vi "test gradient descent.vi"() -> ()   [LabVIEW 2014]
uses:
  Target Functions.ctl
  <vilib>/Analysis/NI_AALBase.lvlib
  <vilib>/vision/Image Controls.llb/IMAQ Image.ctl
  Measurements/Instrument Sequence/Instrument Sequence Notifiers.ctl
  Measurements/Save Data/SaveData Notifiers.ctl
  Autofocus Notifiers.ctl
  Tango XYZ Stage/Tango Notifications.ctl
  Camera/Camera Notifiers.ctl
  Switches and Mirrors/SwitchesMirrors Notifiers.ctl
  NGSLabspec/LabramHR Notifiers.ctl
  Newport ESP301/StressControl Notifiers.ctl
  Keithley707A/Keithley 707A Notifiers.ctl
  HP4155C/HP4155C Notifiers.ctl
  controls/IBM OptoElectroMechanics Message Handler Loop Notifiers.ctl
  support/Notifiers/Notifiers.ctl
  <vilib>/Analysis/Matrix/Datatypes/RealMatrix.ctl
  <vilib>/Analysis/Matrix/NI_Matrix.lvlib
  support/Message Queue/Message Cluster.ctl
  support/Message Queue/IBM OptoElectroMechanics Message Queue.lvlib
  support/Message Queue/All Message Queues.ctl
  Target Refnums.ctl
  AutoFocus Refnums.ctl
  <vilib>/Analysis/baseanly.llb/A x Vector.vi
  ZScan.ctl
panel:
  in  "Z Scan Parameters":T1={"Z Range"=1380.0, "Resolution"=5000.0, "Initial Direction"=enum."Up", "Descent Constant"=0.1} {"Descent Constant" min=0.0 max=1000.0 step=1.0 format="%#_2f"; "Resolution" min=0.0 max=1.0 step=0.01 format="%_2g"; "Z Range" format="%_3g"}
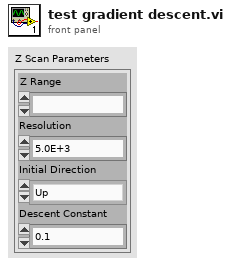
[diagram p1: front panel]
types:
  T1 = typedef "ZScan.ctl" = cluster{"Z Range":ext, "Resolution":dbl, "Initial Direction":enum16{"Up", "Down"}, "Descent Constant":dbl}
  T2 = typedef "AutoFocus Refnums.ctl" = cluster{"Instrument Status":refnum<vi>, "Matching Criteria":refnum<vi>, "Z Scan Parameters":refnum<vi>, "Distance":refnum<vi>, "Transformation Matrix":refnum<vi>, "Match and Edge":T3, "Matching Curves":refnum<vi>, "Tracking":refnum<vi>, "Focus":refnum<vi>, "Find Focus":refnum<vi>, "Set Target":refnum<vi>, "Link Stage & Camera":refnum<vi>, "Align":refnum<vi>}
  T3 = typedef "Target Refnums.ctl" = cluster{"Image":refnum<vi>, "Target":refnum<vi>, "Edge":refnum<vi>, "Target Data":refnum<vi>}
  T4 = typedef "IBM OptoElectroMechanics Message Queue.lvlib/All Message Queues.ctl" = cluster{"Message Handler Loop":refnum<queue>, "Parameter Analyzer":refnum<queue>, "Switching Matrix":refnum<queue>, "Stress Control":refnum<queue>, "Optical Spectrometer":refnum<queue>, "Switches & Mirrors":refnum<queue>, "Camera":refnum<queue>, "XYZ Stage":refnum<queue>, "AutoFocus":refnum<queue>, "Save Data":refnum<queue>, "Plot Data":refnum<queue>, "Instrument Sequence":refnum<queue>, "Strain Measurement":refnum<queue>}
  T5 = typedef "NI_Matrix.lvlib/RealMatrix.ctl" = dbl[][]
  T6 = cluster{"Match":cluster{"Position":cluster{"x":sgl, "y":sgl}, "Angle":sgl, "Scale":sgl, "Score":sgl, "Bounding Box":cluster{"x":sgl, "y":sgl}[]}, "Edge Analysis":cluster{"Mean Value":sgl, "Standard Variation":sgl, "Minimal Value":sgl, "Maximal Value":sgl, "Area (calibrated)":sgl, "Area (pixels)":i32, "%":sgl}}
  T7 = cluster{"Focus Plot":cluster{"Z (um)":dbl[], "Score":sgl[]}[], "max":sgl, "min":sgl}
  T8 = cluster{"Minimum Score":sgl, "Color Score Weight":sgl, "Minimum Contrast":i32, "Match Mode":u32, "Match Feature Mode":u32, "Subpixel Accuracy":bool, "Color Sensitivity":u32, "Search Strategy":u32}
  T9 = typedef "Notifiers.ctl" = cluster{"Message Handler Loop":T10, "Parameter Analyzer":T11, "Switching Matrix":T12, "Stress Control":T13, "Optical Spectrometer":T14, "Switches & Mirrors":T15, "Camera":T16, "XYZ Stage":T17, "AutoFocus":T18, "Save Data":T19, "Plot Data":T19, "Instrument Sequence":T20, "Strain Measurement":cluster{"Status":refnum<notifier>, "Exit":refnum<notifier>, "Ready":refnum<notifier>}}
  T10 = typedef "IBM OptoElectroMechanics Message Handler Loop Notifiers.ctl" = cluster{"Status":refnum<notifier>, "Instrument Data":refnum<notifier>, "Exit":refnum<notifier>, "Ready":refnum<notifier>}
  T11 = typedef "HP4155C Notifiers.ctl" = cluster{"Status":refnum<notifier>, "Instrument Data":refnum<notifier>, "Measurement":refnum<notifier>, "Exit":refnum<notifier>, "Ready":refnum<notifier>}
  T12 = typedef "Keithley 707A Notifiers.ctl" = cluster{"Status":refnum<notifier>, "Instrument Data":refnum<notifier>, "Measurement":refnum<notifier>, "Exit":refnum<notifier>, "Ready":refnum<notifier>}
  T13 = typedef "StressControl Notifiers.ctl" = cluster{"Status":refnum<notifier>, "Instrument Data":refnum<notifier>, "Measurement":refnum<notifier>, "Exit":refnum<notifier>, "Ready":refnum<notifier>}
  T14 = typedef "LabramHR Notifiers.ctl" = cluster{"Status":refnum<notifier>, "Instrument Data":refnum<notifier>, "Measurement":refnum<notifier>, "Exit":refnum<notifier>, "Ready":refnum<notifier>}
  T15 = typedef "SwitchesMirrors Notifiers.ctl" = cluster{"Status":refnum<notifier>, "Instrument Data":refnum<notifier>, "Exit":refnum<notifier>, "Ready":refnum<notifier>}
  T16 = typedef "Camera Notifiers.ctl" = cluster{"Status":refnum<notifier>, "Instrument Data":refnum<notifier>, "Measurement":refnum<notifier>, "Exit":refnum<notifier>, "Ready":refnum<notifier>}
  T17 = typedef "Tango Notifications.ctl" = cluster{"Status":refnum<notifier>, "Instrument Data":refnum<notifier>, "Measurement":refnum<notifier>, "Exit":refnum<notifier>, "Ready":refnum<notifier>}
  T18 = typedef "Autofocus Notifiers.ctl" = cluster{"Status":refnum<notifier>, "Instrument Data":refnum<notifier>, "Measurement":refnum<notifier>, "Exit":refnum<notifier>, "Ready":refnum<notifier>}
  T19 = typedef "SaveData Notifiers.ctl" = cluster{"Status":refnum<notifier>, "Exit":refnum<notifier>, "Ready":refnum<notifier>}
  T20 = typedef "Instrument Sequence Notifiers.ctl" = cluster{"Status":refnum<notifier>, "Instrument Data":refnum<notifier>, "Measurement":refnum<notifier>, "Exit":refnum<notifier>, "Ready":refnum<notifier>}
  T21 = typedef "IMAQ Image.ctl" = refnum<image>
  T22 = typedef "Target Functions.ctl" = enum16{"Setup Match Criteria", "Set Target", "Find Target"}
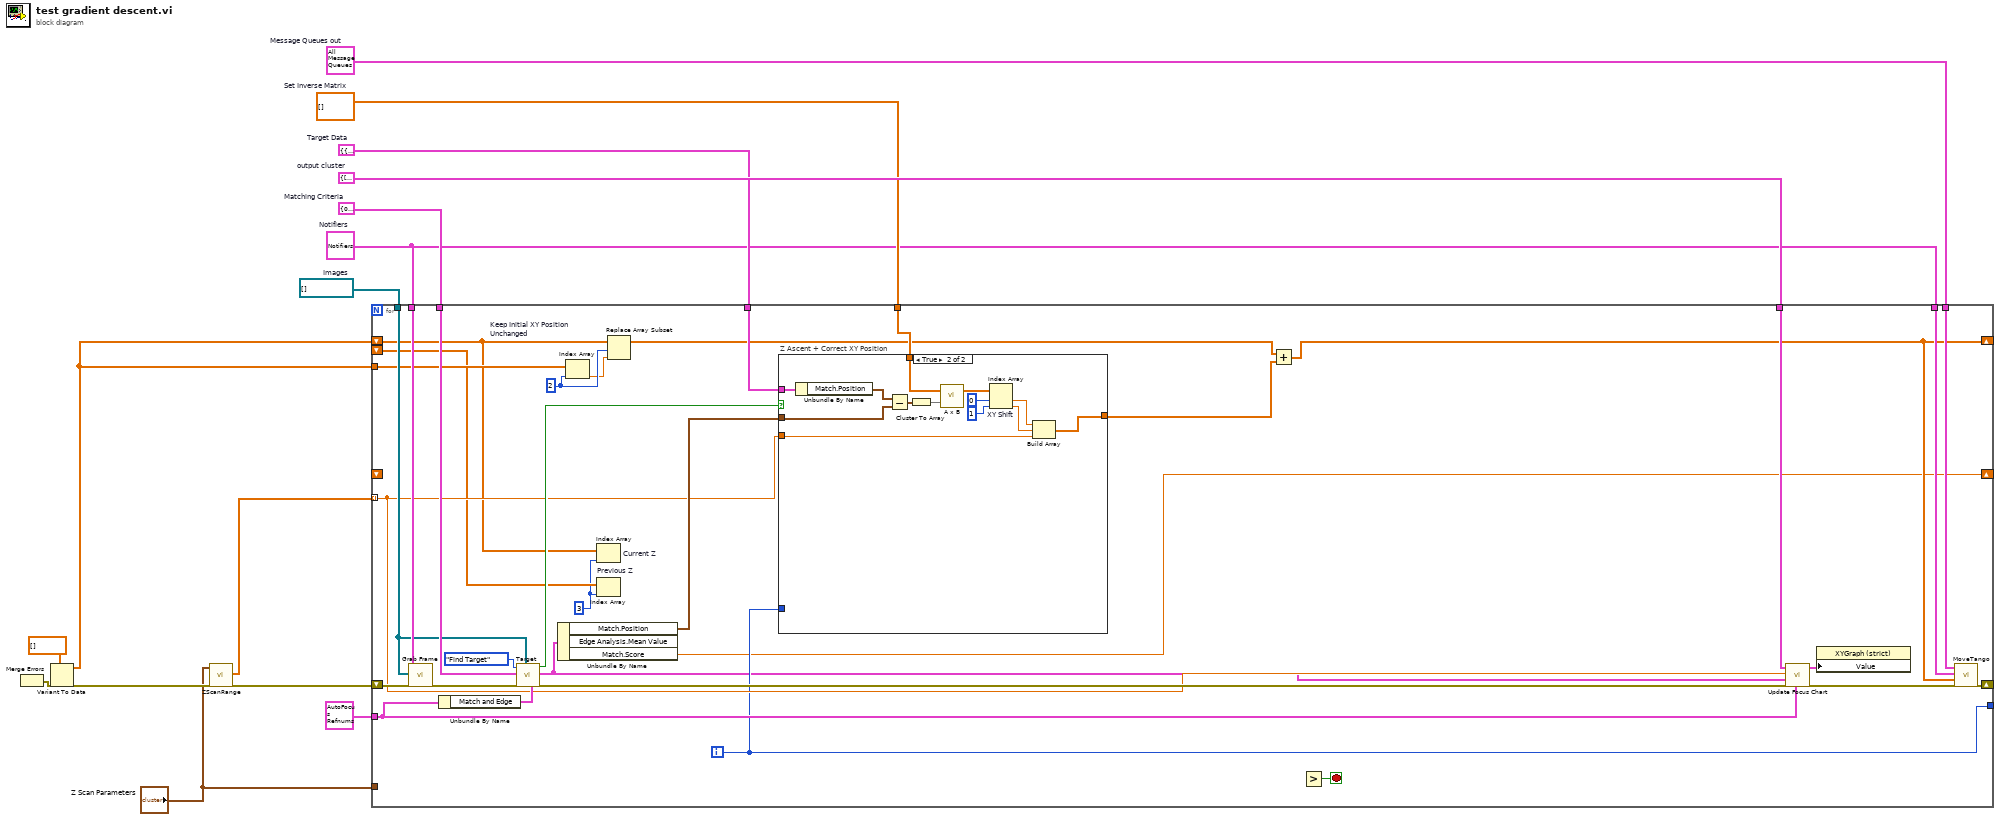
[diagram p0: block diagram]
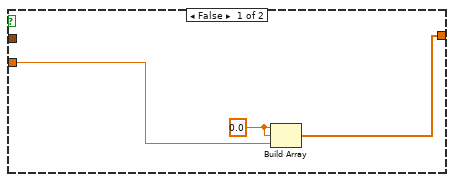
[diagram p2: hidden frame]
diagram:
  w3 = T4 {"Message Handler Loop"=refnum, "Parameter Analyzer"=refnum, "Switching Matrix"=refnum, "Stress Control"=refnum, "Optical Spectrometer"=refnum, "Switches & Mirrors"=refnum, "Camera"=refnum, "XYZ Stage"=refnum, "AutoFocus"=refnum, "Save Data"=refnum, "Plot Data"=refnum, "Instrument Sequence"=refnum, "Strain Measurement"=refnum}  # Message Queues out
  w4 = T5 []  # Set Inverse Matrix
  w5 = T6 {"Match"={"Position"={"x"=0.0, "y"=0.0}, "Angle"=0.0, "Scale"=0.0, "Score"=0.0, "Bounding Box"=[]}, "Edge Analysis"={"Mean Value"=0.0, "Standard Variation"=0.0, "Minimal Value"=0.0, "Maximal Value"=0.0, "Area (calibrated)"=0.0, "Area (pixels)"=0, "%"=0.0}}  # Target Data
  w6 = T7 {"Focus Plot"=[], "max"=0.0, "min"=0.0}  # output cluster
  w7 = T8 {"Minimum Score"=0.0, "Color Score Weight"=0.0, "Minimum Contrast"=0, "Match Mode"=0, "Match Feature Mode"=0, "Subpixel Accuracy"=FALSE, "Color Sensitivity"=0, "Search Strategy"=0}  # Matching Criteria
  w1 = T9 {"Message Handler Loop"={"Status"=refnum, "Instrument Data"=refnum, "Exit"=refnum, "Ready"=refnum}, "Parameter Analyzer"={"Status"=refnum, "Instrument Data"=refnum, "Measurement"=refnum, "Exit"=refnum, "Ready"=refnum}, "Switching Matrix"={"Status"=refnum, "Instrument Data"=refnum, "Measurement"=refnum, "Exit"=refnum, "Ready"=refnum}, "Stress Control"={"Status"=refnum, "Instrument Data"=refnum, "Measurement"=refnum, "Exit"=refnum, "Ready"=refnum}, "Optical Spectrometer"={"Status"=refnum, "Instrument Data"=refnum, "Measurement"=refnum, "Exit"=refnum, "Ready"=refnum}, "Switches & Mirrors"={"Status"=refnum, "Instrument Data"=refnum, "Exit"=refnum, "Ready"=refnum}, "Camera"={"Status"=refnum, "Instrument Data"=refnum, "Measurement"=refnum, "Exit"=refnum, "Ready"=refnum}, "XYZ Stage"={"Status"=refnum, "Instrument Data"=refnum, "Measurement"=refnum, "Exit"=refnum, "Ready"=refnum}, "AutoFocus"={"Status"=refnum, "Instrument Data"=refnum, "Measurement"=refnum, "Exit"=refnum, "Ready"=refnum}, "Save Data"={"Status"=refnum, "Exit"=refnum, "Ready"=refnum}, "Plot Data"={"Status"=refnum, "Exit"=refnum, "Ready"=refnum}, "Instrument Sequence"={"Status"=refnum, "Instrument Data"=refnum, "Measurement"=refnum, "Exit"=refnum, "Ready"=refnum}, "Strain Measurement"={"Status"=refnum, "Exit"=refnum, "Ready"=refnum}}  # Notifiers
  w8 = T21[] []  # Images
  n1 = Merge Errors() -> (w15:errorcluster)  [unwired: 2 in]
  n2 = Variant To Data(error in=w15, type=dbl[] [] ("PosOut")) -> (data=w10:dbl[], error out=w13:errorcluster)  [unwired: 1 in]
  n3 = call "ZScanRange.vi"("error in (no error)"=w13, "Z Scan Parameters"="Z Scan Parameters") -> ("error out"=w12:errorcluster, "Displacements"=w11:dbl[])  [unwired: 8 in]
  n4 = for {
    tunnel: w8 -> [w43]
    tunnel: w7 -> [w46]
    tunnel: T2 {"Instrument Status"=refnum, "Matching Criteria"=refnum, "Z Scan Parameters"=refnum, "Distance"=refnum, "Transformation Matrix"=refnum, "Match and Edge"={"Image"=refnum, "Target"=refnum, "Edge"=refnum, "Target Data"=refnum}, "Matching Curves"=refnum, "Tracking"=refnum, "Focus"=refnum, "Find Focus"=refnum, "Set Target"=refnum, "Link Stage & Camera"=refnum, "Align"=refnum} ("Refnums") -> [w42]
    shift-right: [w29] -> _
    shift-left: w12 -> [w33]
    tunnel: w1 -> [w44]
    tunnel: w11 -> [w23] mode=indexing
    tunnel: w6 -> [w39]
    tunnel: w5 -> [w36]
    tunnel: [w20] -> _
    tunnel: w4 -> [w34]
    tunnel: w1 -> [w32]
    tunnel: w3 -> [w31]
    shift-right: [w28] -> _
    shift-left: w10 -> [w21]
    tunnel: w10 -> [w26]
    tunnel: "Z Scan Parameters" -> [_]
    shift-right: [w16] -> _
    shift-left: _ -> [_]
    shift-left: _ -> [w19]
    i -> [w20]
    stop <- w40 stop-if-true
    w18 = 3 ("index")
    w25 = 2 ("index")
    n5 = call "Grab Frame.vi"("error in (no error)"=w33, "Images"=w43, "Notifiers"=w44) -> ("error out"=w45:errorcluster)  [unwired: 7 in, 1 out]
    n6 = Unbundle By Name(w42) -> ("Match and Edge"=w48:T3)
    n7 = call "Target.vi"("Refnums"=w48, "Images"=w43, "error in (no error)"=w45, "Pattern Matching Criteria"=w46, "Function"=Target_Functions."Find Target") -> ("error out"=w41:errorcluster, "Target Data"=w17:T6, "Target Found?"=w35:bool)  [unwired: 4 in]
    n8 = Unbundle By Name(w17) -> ("Match.Position"=w37:cluster{"x":sgl, "y":sgl}, "Match.Score"=w16:sgl)  [unwired: 1 out]
    n9 = Index Array(array=w26, index=w25) -> (element=w24:dbl)
    n10 = Index Array "Current Z"(array=w21, index=w18) -> ()  [unwired: 1 out]
    n11 = Index Array "Previous Z"(array=w19, index=w18) -> ()  [unwired: 1 out]
    n12 = Replace Array Subset "Keep Initial XY Position Unchanged"(array=w21, new element=w24, index=w25) -> (w27:dbl[])
    n13 = case "Z Ascent + Correct XY Position" shown="True" w35 {
      tunnel: w37 -> [_ w56]
      tunnel: w36 -> [_ w59]
      tunnel: w34 -> [_ w58]
      tunnel: [w49 w53] -> w22
      tunnel: w23 -> [w51 w52]
      tunnel: w20 -> [_ _]
      frame False {
        w50 = 0.0
        n14 = Build Array(w50, w50, w51) -> (w49:dbl[])
      }
      frame True {
        n15 = Unbundle By Name(w59) -> ("Match.Position"=w57:cluster{"x":sgl, "y":sgl})
        n16 = Subtract(x=w57, y=w56) -> (x-y=w61:cluster{"x":sgl, "y":sgl})
        n17 = Cluster To Array(cluster=w61) -> (array=w60:sgl[])
        n18 = call-poly <vilib>:"A x B.vi"("Vector"=w60, "A"=w58) -> ("A x Vector"=w64:dbl[])  [unwired: 1 out]
        n19 = Index Array "XY Shift"(array=w64, index #1=0 ("index"), index #2=1 ("index")) -> (element #1=w55:dbl, element #2=w54:dbl)
        n20 = Build Array(w55, w54, w52) -> (w53:dbl[])
      }
    }
    n21 = Add(x=w27, y=w22) -> (x+y=w28:dbl[])
    n22 = Greater?() -> (0:w40:bool)  [unwired: 2 in]
    n23 = call "Update Focus Chart.vi"("Refnums"=w42, "error in (no error)"=w41, "Target Data"=w17, "Numeric"=w23, "output cluster"=w39) -> ("error out"=w30:errorcluster, "Focus Plot"=w38:cluster{"Z (um)":dbl[], "Score":sgl[]}[])  [unwired: 5 in]
    n24 = property on="Property Node" class="XYGraph (strict)"("Value"=w38) -> ()  [unwired: 2 in, 2 out]
    n25 = call "MoveTango.vi"("error in (no error)"=w30, "Destination coordinate"=w28, "Notifiers"=w32, "Message Queues in"=w31) -> ("error out"=w29:errorcluster)  [unwired: 7 in]
  }
